vi "Set Custom Symbol.vi"(8 "error in":errorcluster, 10 "Symbol File Path":path) -> (0 "error out":errorcluster)   [LabVIEW 2026, in "Tree Map.lvlib" / "Tree Map.lvclass"]
uses:
  Tree Map.lvclass
panel:
  out "Index":i32
  in  "Tree":refnum<vi>
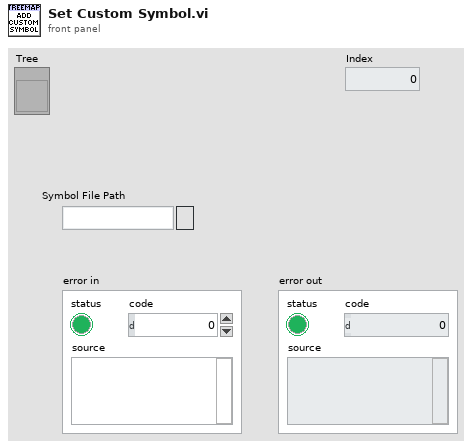
[diagram p1: front panel]
types:
  T1 = cluster{"image type":i32, "image depth":i32, "image":u8[], "mask":u8[], "colors":u32[], "Rectangle":cluster{"left":i16, "top":i16, "right":i16, "bottom":i16}}[]
  T2 = typedef "imagedata.ctl" = cluster{"image type":i32, "image depth":i32, "image":u8[], "mask":u8[], "colors":u32[], "Rectangle":cluster{"left":i16, "top":i16, "right":i16, "bottom":i16}}
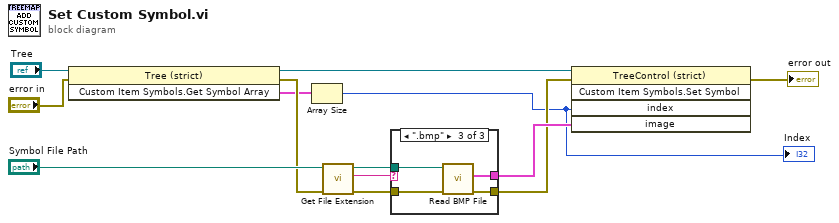
[diagram p0: block diagram]
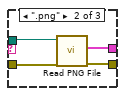
[diagram p3: hidden frame]
diagram:
  n1 = invoke class="Tree (strict)" method="Custom Item Symbols.Get Symbol Array"(reference="Tree", error in="error in") -> (reference out=w5:refnum<vi>, error out=w7:errorcluster, "Custom Glyphs:Get Glyph Array"=w6:T1)  [unwired: 1 in]
  n2 = Array Size(array=w6) -> (size(s)=w1:i32)
  "Index" <- w1
  n3 = call <vilib>:"Get File Extension.vi"("error in (no error)"=w7, "file"="Symbol File Path") -> ("error out"=w10:errorcluster, "lowercase file extension"=w12:string, "dup file"=w11:path)  [unwired: 5 in, 2 out]
  n4 = case shown="\".bmp\"" w12 {
    tunnel: w11 -> [_ w15 w22]
    tunnel: w10 -> [w14 w18 w21]
    tunnel: [_ w16 w20] -> w4
    tunnel: [w14 w17 w19] -> w3
    frame Default {
    }
    frame ".png" {
      n5 = call <vilib>:"Read PNG File.vi"("error in (no error)"=w18, "path to PNG file"=w15) -> ("error out"=w17:errorcluster, "image data"=w16:T2)  [unwired: 7 in, 1 out]
    }
    frame ".bmp" {
      n6 = call <vilib>:"Read BMP File.vi"("error in (no error)"=w21, "path to BMP file"=w22) -> ("error out"=w19:errorcluster, "image data"=w20:T2)  [unwired: 7 in, 1 out]
    }
  }
  n7 = invoke on="Invoke Node" class="TreeControl (strict)" method="Custom Item Symbols.Set Symbol"(reference=w5, error in=w3, "index"=w1, "image"=w4) -> (error out=→"error out":errorcluster)  [unwired: 1 in, 4 out]
